vi "Generate PDF.vi"(8 "error in":errorcluster, 10 "Dynamic report parameters":T2, 11 "ZenReport private":T1) -> (0 "error out":errorcluster, 2 "Detailed error out":string, 3 "ZenReport private data":T1)   [LabVIEW 2015]
uses:
  Typedefs/Dynamic report parameters.ctl
  Typedefs/ZenReport private.ctl
  Typedefs/Report generation data cluster (internal use).ctl
  <vilib>/vision/Image Controls.llb/IMAQ Image.ctl
  <userlib>/_OpenG.lib/file/file.llb/Valid Path - Traditional__ogtk.vi
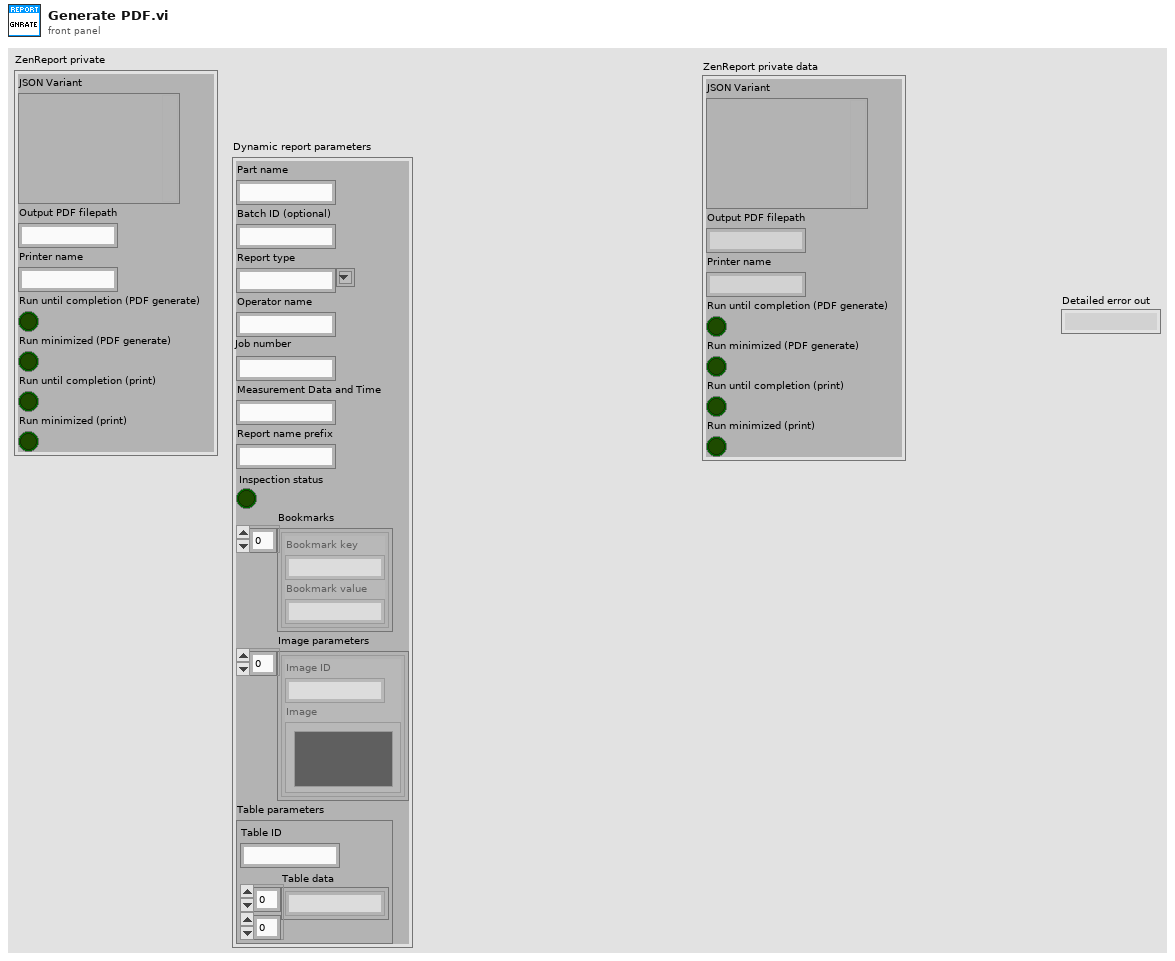
[diagram p1: front panel]
types:
  T1 = typedef "ZenReport private.ctl" = cluster{"JSON Variant":variant, "Output PDF filepath":string, "Printer name":string, "Run until completion (PDF generate)":bool, "Run minimized (PDF generate)":bool, "Run until completion (print)":bool, "Run minimized (print)":bool}
  T2 = typedef "Dynamic report parameters.ctl" = cluster{"Part name":string, "Batch ID (optional)":string, "Report type":string, "Operator name":string, "Job number":string, "Measurement Data and Time":string, "Report name prefix":string, "Inspection status":bool, "Bookmarks":cluster{"Bookmark key":string, "Bookmark value":string}[], "Image parameters":cluster{"Image ID":string, "Image":T3}[], "Table parameters":cluster{"Table ID":string, "Table data":string[][]}}
  T3 = typedef "IMAQ Image.ctl" = refnum<image>
  T4 = typedef "Report generation data cluster (internal use).ctl" = cluster{"Report data":cluster{"$part_name$":string, "$batch_id$":string, "$customer_name$":string, "$operator_name$":string, "$system_name$":string, "$measurement_date_and_time$":string, "$location$":string, "$job_number$":string, "$department$":string, "$status$":string, "Table details":string[][], "Output PDF filepath":string, "Output PDF folder filepath":path}, "Image details":cluster{"Image":T3, "Image filepath":path, "Use default scaling":bool, "Image scaling":cluster{"$image_width$":u32, "$image_height$":u32, "Unit":string}, "Resample factor":dbl}, "Report parameters":cluster{"Report auto name":bool, "Name prefix":string, "Printer name":string}}
  T5 = typedef "ZenReport internal data.ctl" = cluster{"ZenReport configuration":cluster{"System configuration":T6, "Part configuration":T7, "Batch parameters":T8}, "Report private parameters":T9}
  T6 = typedef "System configuration.ctl" = cluster{"System based configuration":cluster{"SystemName":string, "CompanyName":string, "Location":string, "Department":string, "LogoFilepath":string, "ImageTempFilePath":string, "PrinterParameters":cluster{"PrinterNamesList":string[], "DefaultPrinterName":string}}}
  T7 = typedef "Part configuration.ctl" = cluster{"Part configuration":cluster{"ReportType":string, "TableParameters":cluster{"TableID":dbl, "Column details":cluster{"ColumnName":string, "ColumnWidth":dbl, "ColumnTextAlignment":string}[]}[], "ImageParameters":cluster{"ImageID":string, "ImageBookmark":string, "ImageScalingParameters":cluster{"Width":u32, "Height":u32, "Unit":string}, "DefaultDisplayString":string, "ImageFilepath":string, "ResamplingFactor":dbl, "UseDefaultScaling":bool}[], "OutputReportNamePrefix":string, "OutputFilePath":string, "DefaultBookmarkValues":cluster{"BookmarkKey":string, "BookmarkValue":string}[]}}
  T8 = typedef "Batch configuration.ctl" = cluster{"Batch parameters":cluster{"ReportType":string, "TableParameters":cluster{"TableID":dbl, "Column details":cluster{"ColumnName":string, "ColumnWidth":dbl, "ColumnTextAlignment":string}[]}[], "OutputReportNamePrefix":string, "OutputFilePath":string, "ImageParameters":cluster{"ImageID":string, "ImageBookmark":string, "ImageScalingParameters":cluster{"Width":u32, "Height":u32, "Unit":string}, "DefaultDisplayString":string, "ImageFilepath":string, "ResamplingFactor":dbl, "UseDefaultScaling":bool}[]}}
  T9 = typedef "Internal data.ctl" = cluster{"Tex string":string}
  T10 = cluster{"ImageID":string, "ImageBookmark":string, "ImageScalingParameters":cluster{"Width":u32, "Height":u32, "Unit":string}, "DefaultDisplayString":string, "ImageFilepath":string, "ResamplingFactor":dbl, "UseDefaultScaling":bool}[]
  T11 = cluster{"ImageID":string, "ImageBookmark":string, "ImageScalingParameters":cluster{"Width":u32, "Height":u32, "Unit":string}, "DefaultDisplayString":string, "ImageFilepath":string, "ResamplingFactor":dbl, "UseDefaultScaling":bool}
  T12 = cluster{"Image":T3, "Image filepath":path, "Use default scaling":bool, "Image scaling":cluster{"$image_width$":u32, "$image_height$":u32, "Unit":string}, "Resample factor":dbl}
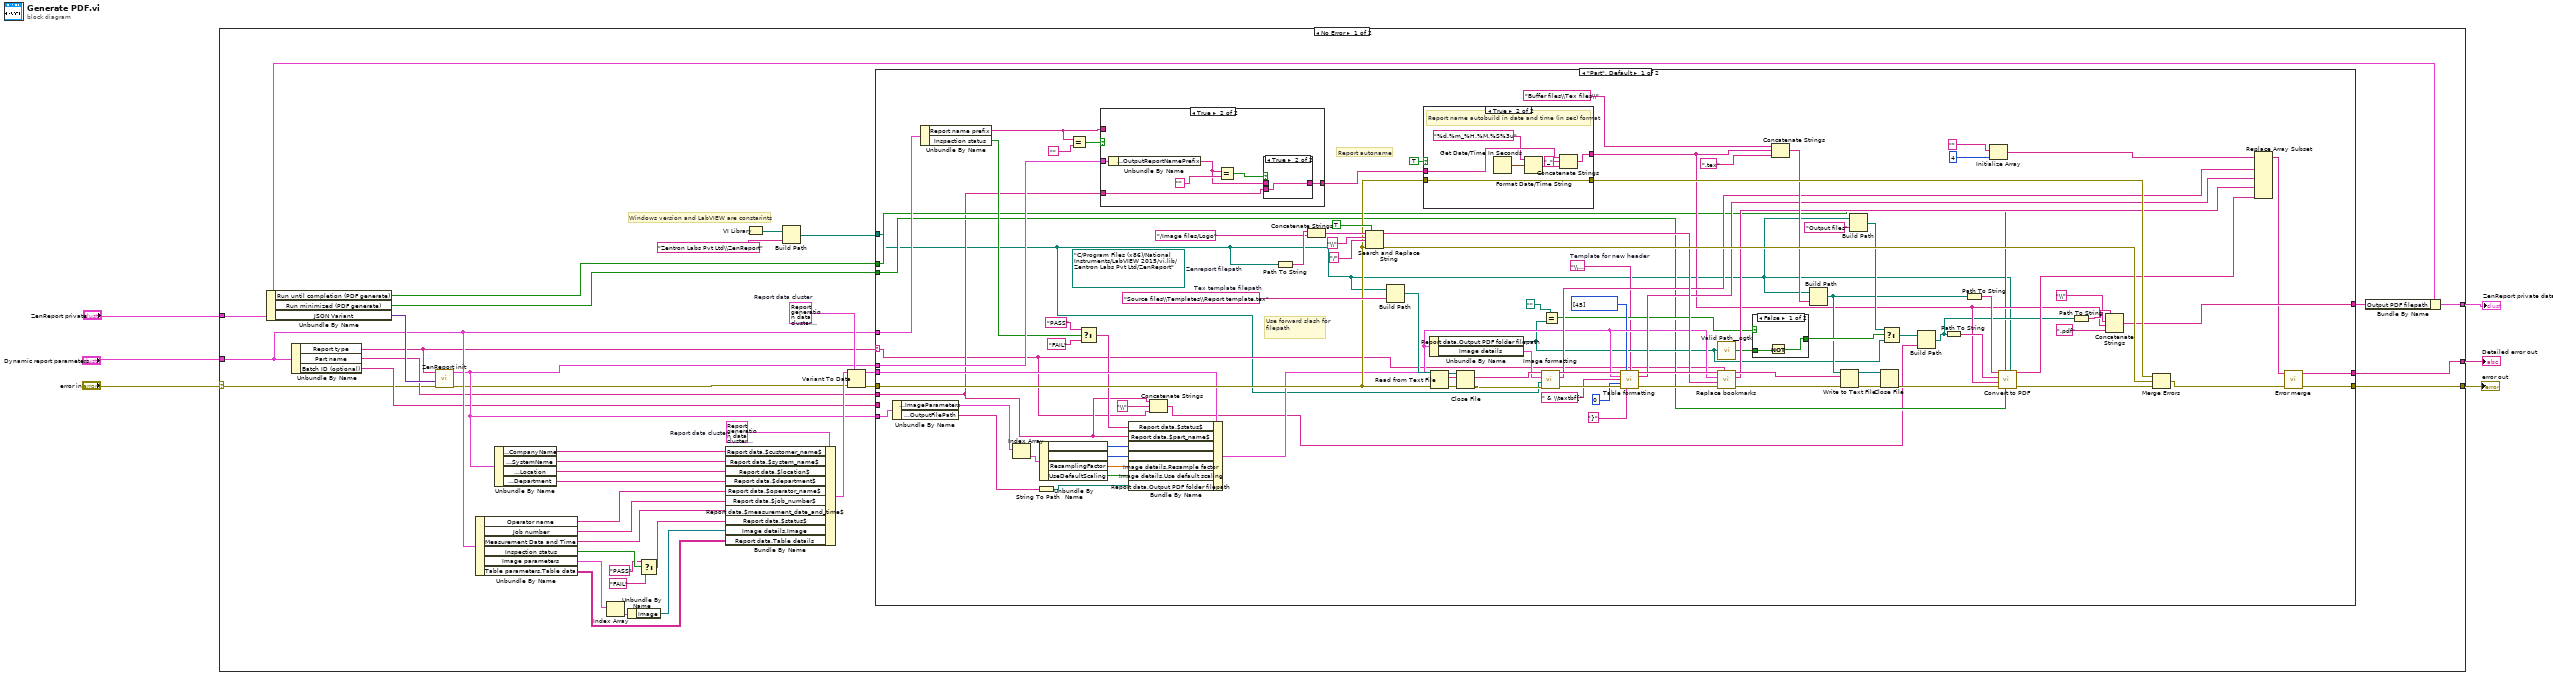
[diagram p0: block diagram]
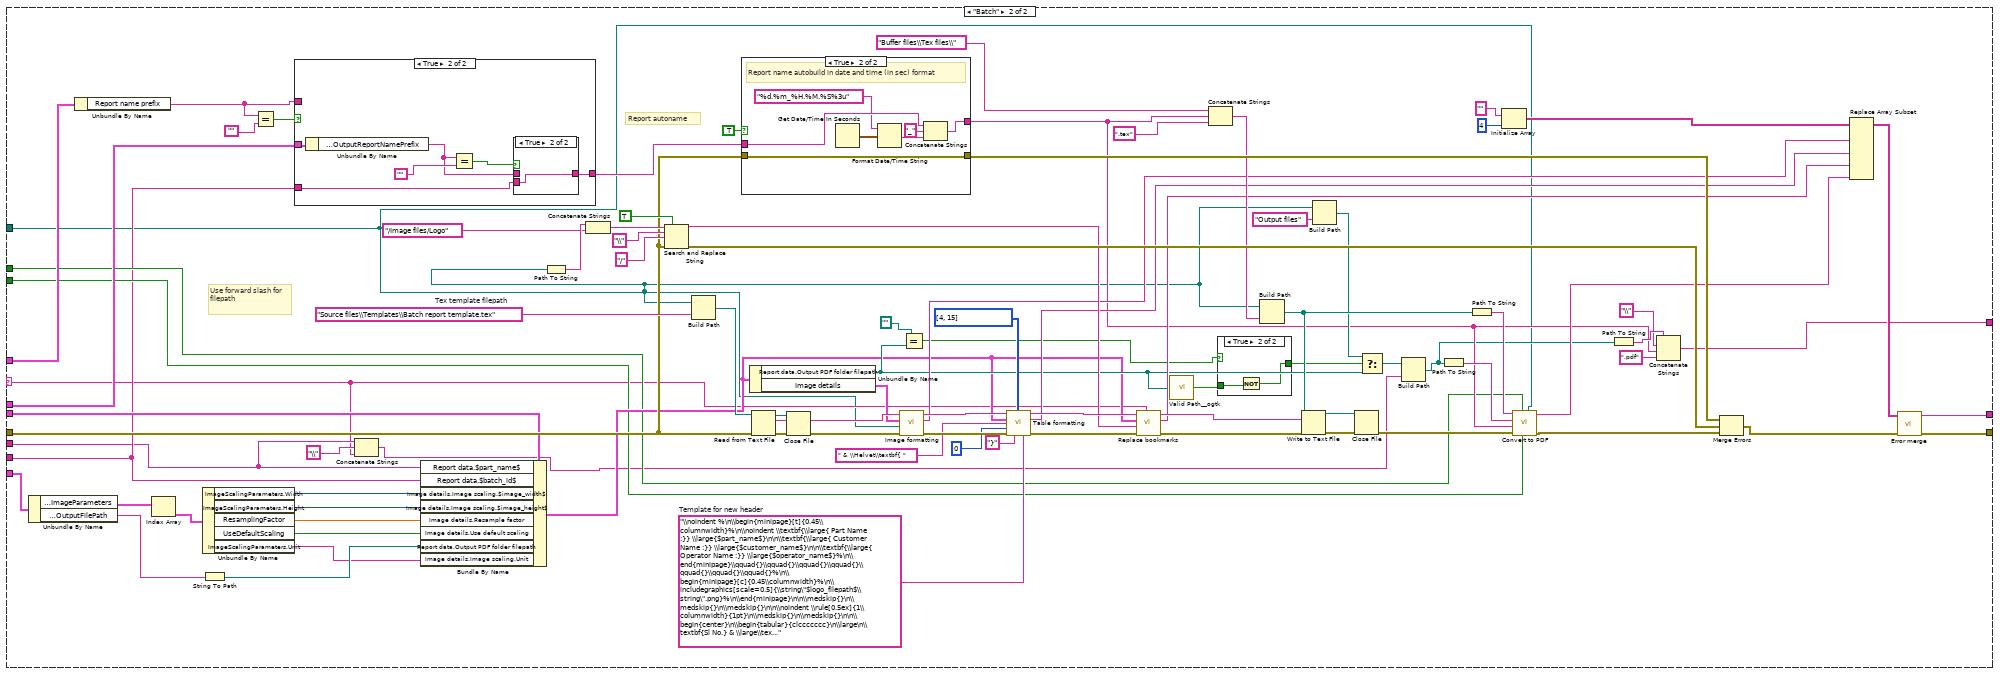
[diagram p6: hidden frame]
diagram:
  n1 = case shown="No Error" "error in" {
    selector: "error in" -> [w9 w267]
    tunnel: [w44 w267] -> w6
    tunnel: "Dynamic report parameters" -> [w25 _]
    tunnel: "ZenReport private" -> [w22 _]
    tunnel: [w11 _] -> w3
    tunnel: [w10 _] -> w2
    frame No Error {
      w27 = T4 {"Report data"={"$part_name$"="", "$batch_id$"="", "$customer_name$"="", "$operator_name$"="", "$system_name$"="", "$measurement_date_and_time$"="", "$location$"="", "$job_number$"="", "$department$"="", "$status$"="", "Table details"=[], "Output PDF filepath"="", "Output PDF folder filepath"=path ""}, "Image details"={"Image"=refnum, "Image filepath"=path "", "Use default scaling"=TRUE, "Image scaling"={"$image_width$"=0, "$image_height$"=0, "Unit"="mm"}, "Resample factor"=0.0}, "Report parameters"={"Report auto name"=FALSE, "Name prefix"="", "Printer name"=""}}  # Report data cluster
      w28 = T4 {"Report data"={"$part_name$"="", "$batch_id$"="", "$customer_name$"="", "$operator_name$"="", "$system_name$"="", "$measurement_date_and_time$"="", "$location$"="", "$job_number$"="", "$department$"="", "$status$"="", "Table details"=[], "Output PDF filepath"="", "Output PDF folder filepath"=path ""}, "Image details"={"Image"=refnum, "Image filepath"=path "", "Use default scaling"=TRUE, "Image scaling"={"$image_width$"=0, "$image_height$"=0, "Unit"="mm"}, "Resample factor"=0.0}, "Report parameters"={"Report auto name"=FALSE, "Name prefix"="", "Printer name"=""}}  # Report data cluster
      # "Windows version and LabVIEW are constarints"
      n2 = Unbundle By Name(w22) -> ("Run until completion (PDF generate)"=w15:bool, "Run minimized (PDF generate)"=w14:bool, "JSON Variant"=w43:variant)
      n3 = Unbundle By Name(w25) -> ("Report type"=w12:string, "Part name"=w13:string, "Batch ID (optional)"=w19:string)
      n4 = call "ZenReport init.vi"("error IO"=w9, "Get part / batch data"=w43, "Report type"=w12) -> ("Error out"=w8:errorcluster, "output cluster"=w20:T5)  [unwired: 7 in]
      n5 = Unbundle By Name(w25) -> ("Operator name"=w33:string, "Job number"=w34:string, "Measurement Data and Time"=w38:string, "Inspection status"=w37:bool, "Image parameters"=w40:cluster{"Image ID":string, "Image":T3}[], "Table parameters.Table data"=w7:string[][])
      n6 = Unbundle By Name(w20) -> ("ZenReport configuration.System configuration.System based configuration.CompanyName"=w29:string, "ZenReport configuration.System configuration.System based configuration.SystemName"=w30:string, "ZenReport configuration.System configuration.System based configuration.Location"=w31:string, "ZenReport configuration.System configuration.System based configuration.Department"=w32:string)
      n7 = Index Array(array=w40) -> (element=w41:cluster{"Image ID":string, "Image":T3})  [unwired: 1 in]
      n8 = Unbundle By Name(w41) -> ("Image"=w42:T3)
      n9 = Select(t="PASS", s=w37, f="FAIL") -> (s? t:f=w39:string)
      n10 = Bundle By Name(cluster=w28, "Report data.$customer_name$"=w29, "Report data.$system_name$"=w30, "Report data.$location$"=w31, "Report data.$department$"=w32, "Report data.$operator_name$"=w33, "Report data.$job_number$"=w34, "Report data.$measurement_date_and_time$"=w38, "Report data.$status$"=w39, "Image details.Image"=w42, "Report data.Table details"=w7) -> (w26:T4)
      n11 = VI Library() -> (path=w18:path)
      n12 = Build Path(base path=w18, name or relative path="Zentron Labs Pvt Ltd\\ZenReport") -> (appended path=w16:path)
      n13 = Variant To Data(error in=w8, type=w27, Variant=w26) -> (data=w23:T4, error out=w24:errorcluster)
      n14 = case shown="\"Part\", Default" w12 {
        selector: w12 -> [w47 w159]
        tunnel: [w51 w163] -> w44
        tunnel: [w91 w199] -> w10
        tunnel: w24 -> [w89 w196]
        tunnel: w20 -> [w64 w193]
        tunnel: w25 -> [w63 w173]
        tunnel: w16 -> [w45 w157]
        tunnel: w23 -> [w80 w175]
        tunnel: [w88 w192] -> w21
        tunnel: w20 -> [w76 w189]
        tunnel: w13 -> [w48 w161]
        tunnel: w19 -> [_ w162]
        tunnel: w15 -> [w53 w165]
        tunnel: w14 -> [w52 w164]
        frame "Part", Default {
          w61 = "\\noindent %\n\\begin{minipage}[t]{0.45\\columnwidth}%\n\\noindent \\textbf{Part Name : $part_name$}\n\n\\textbf{Customer Name : $customer_name$}\n\n\\textbf{Operator Name : $operator_name$}%\n\\end{minipage}\\qquad{}\\qquad{}\\qquad{}\\qquad{}\\qquad{}\\qquad{}\\qquad{}%\n\\begin{minipage}[c]{0.45\\columnwidth}%\n\\includegraphics[scale=0.5]{\\string\"$logo_filepath$\\string\".png}%\n\\end{minipage}\n\n\\medskip{}\n\\medskip{}\n\\medskip{}\n\n\\noindent \\rule[0.5ex]{1\\columnwidth}{1pt}\n\n\\begin{center}\n\\begin{tabular}{clccccccc}\n\\textbf{SL.NO} & \\textbf{DESCRIPTION} & \\textbf{LSL} & \\textbf{NOMINAL} & \\textbf{USL} & \\textbf{MEASURED} & \\textbf{DEVIATION} & \\textbf{UNITS} & \\textbf{STATUS}\\tabularnewline\n &  &  &  &  &  &  &  & \\tabularnewline\n$table2$\n\\end{tabular}\n\\end{center}\n\n\\end{document}\n"  # Template for new header
          (unwired) path "C:/Program Files (x86)/National Instruments/LabVIEW 2015/vi.lib/Zentron Labs Pvt Ltd/ZenReport"  # Zenreport filepath
          w135 = "Source files\\Templates\\Report template.tex"  # Tex template filepath
          # "Report autoname"
          # "Use forward slash for filepath"
          n15 = Unbundle By Name(w76) -> ("ZenReport configuration.Part configuration.Part configuration.ImageParameters"=w75:T10, "ZenReport configuration.Part configuration.Part configuration.OutputFilePath"=w73:string)
          n16 = Unbundle By Name(w63) -> ("Report name prefix"=w65:string, "Inspection status"=w58:bool)
          n17 = Index Array(array=w75) -> (element=w84:T11)  [unwired: 1 in]
          n18 = String To Path(string=w73) -> (path=w74:path)
          n19 = Unbundle By Name(w84) -> ("ImageScalingParameters.Width"=w83:u32, "ImageScalingParameters.Height"=w82:u32, "ResamplingFactor"=w81:dbl, "UseDefaultScaling"=w78:bool)
          n20 = Equal?(x=w65, y="") -> (x = y?=w66:bool)
          n21 = Select(t="PASS", s=w58, f="FAIL") -> (s? t:f=w57:string)
          n22 = case shown="True" w66 {
            tunnel: [w136 w140] -> w62
            tunnel: w64 -> [_ w138]
            tunnel: w48 -> [_ w137]
            tunnel: w65 -> [w136 _]
            frame False {
            }
            frame True {
              n23 = Unbundle By Name(w138) -> ("ZenReport configuration.Part configuration.Part configuration.OutputReportNamePrefix"=w139:string)
              n24 = Equal?(x=w139, y="") -> (x = y?=w141:bool)
              n25 = case shown="True" w141 {
                tunnel: [w143 w144] -> w140
                tunnel: w139 -> [w143 _]
                tunnel: w137 -> [_ w144]
                frame False {
                }
                frame True {
                }
              }
            }
          }
          n26 = Bundle By Name(cluster=w80, "Report data.$status$"=w57, "Report data.$part_name$"=w48, "Image details.Image scaling.$image_width$"=w83, "Image details.Image scaling.$image_height$"=w82, "Image details.Resample factor"=w81, "Image details.Use default scaling"=w78, "Report data.Output PDF folder filepath"=w74) -> (w79:T4)
          n27 = Concatenate Strings(w48, "\\" ("string"), w47) -> (w46:string)
          n28 = Path To String(path=w45) -> (string=w129:string)
          n29 = Concatenate Strings(w129, "/Image files/Logo") -> (w127:string)
          n30 = Search and Replace String(replace all?=TRUE ("replace all? (F)"), input string=w127, search string="\\", replace string="/" ("replace string (\"\")"), error in=w89) -> (result string=w106:string, error out=w123:errorcluster)  [unwired: 3 in, 2 out]
          n31 = Build Path(base path=w45, name or relative path=w135) -> (appended path=w134:path)
          n32 = case shown="True" TRUE {
            tunnel: w62 -> [w149 w154]
            tunnel: [w149 w155] -> w56
            tunnel: w89 -> [w148 w152]
            tunnel: [w148 w152] -> w119
            frame False {
              # "Write in given name"
            }
            frame True {
              # "Report name autobuild in date and time (in sec) format"
              n33 = Get Date/Time In Seconds() -> (seconds since 1Jan1904=w156:timestamp)
              n34 = Format Date/Time String(time format string (%c)="%d.%m_%H.%M.%S%3u", seconds (now)=w156) -> (date/time string=w150:string)  [unwired: 1 in]
              n35 = Concatenate Strings(w154, "_" ("string"), w150) -> (w155:string)
            }
          }
          n36 = Unbundle By Name(w79) -> ("Report data.Output PDF folder filepath"=w68:path, "Image details"=w112:T12)
          n37 = Read from Text File(file (use dialog)=w134, error in=w89) -> (refnum out=w131:refnum<file>, text=w113:string, error out=w132:errorcluster)  [unwired: 2 in, 1 out]
          n38 = Close File(refnum=w131, error in=w132) -> (error out=w114:errorcluster)  [unwired: 1 out]
          n39 = call "Image formatting.vi"("error in (no error)"=w114, "Zenreport filepath"=w45, "Image details"=w112, "Tex string in"=w113) -> ("error out"=w122:errorcluster, "Error details out"=w94:string, "Tex string out"=w111:string)  [unwired: 5 in]
          n40 = Equal?(x=path "", y=w68) -> (x = y?=w72:bool)
          n41 = call "Table formatting.vi"("Input tex string"=w111, "Table row count array"=i32[] [45], "Template for new header"=w61, "Report data cluster"=w79, "Separator"=" & \\textbf{", "Iteration count"=u8 0, "error in (no error)"=w122, "End tag"="}") -> ("Tex string out"=w108:string, "Error details out"=w93:string, "error out"=w110:errorcluster)  [unwired: 5 in]
          n42 = call "Replace bookmarks.vi"("Report type"=w47, "error in (no error)"=w110, "Logo filepath"=w106, "Report data cluster"=w79, "Tex file string"=w108) -> ("error out"=w109:errorcluster, "Error detail out"=w92:string, "Tex file string out"=w107:string)  [unwired: 4 in]
          n43 = call-poly <userlib>:"Valid Path__ogtk.vi"("path"=w68) -> ("valid"=w71:bool)
          n44 = case shown="False" w72 {
            selector: w72 -> [_ w147]
            tunnel: w71 -> [w146 _]
            tunnel: [w145 w147] -> w70
            frame False {
              n45 = Not(x=w146) -> (.not. x?=w145:bool)
            }
            frame True {
            }
          }
          n46 = Concatenate Strings("Buffer files\\Tex files\\" ("string"), w56, ".tex" ("string")) -> (w118:string)
          n47 = Build Path(base path=w45, name or relative path=w118) -> (appended path=w69:path)
          n48 = Write to Text File(file (use dialog)=w69, text=w107, error in=w109) -> (refnum out=w130:refnum<file>, error out=w133:errorcluster)  [unwired: 1 in, 1 out]
          n49 = Build Path(base path=w45, name or relative path="Output files") -> (appended path=w100:path)
          n50 = Close File(refnum=w130, error in=w133) -> (error out=w105:errorcluster)  [unwired: 1 out]
          n51 = Select(t=w100, s=w70, f=w68) -> (s? t:f=w55:path)
          n52 = Build Path(base path=w55, name or relative path=w46) -> (appended path=w54:path)
          n53 = Path To String(path=w54) -> (string=w99:string)
          n54 = Path To String(path=w69) -> (string=w103:string)
          n55 = Initialize Array("", 4 ("dimension size")) -> (w96:string[])
          n56 = call "Convert to PDF.vi"("Zenreport filepath"=w45, "run minimized? (F)"=w52, "wait until completion? (T)"=w53, "error in"=w105, "PDF name"=w56, "Destination filepath"=w99, "Source filepath"=w103) -> ("error out"=w104:errorcluster, "Error detail out"=w95:string)  [unwired: 3 in]
          n57 = Path To String(path=w54) -> (string=w116:string)
          n58 = Concatenate Strings(w116, "\\" ("string"), w56, ".pdf" ("string")) -> (w88:string)
          n59 = Merge Errors(w119, w123, w104) -> (w51:errorcluster)
          n60 = Replace Array Subset(array=w96, new element #1=w94, new element #2=w93, new element #3=w92, new element #4=w95) -> (w50:string[])  [unwired: 4 in]
          n61 = call "Error merge.vi"("Error details array"=w50) -> ("Detailed error out"=w91:string)  [unwired: 10 in]
        }
        frame "Batch" {
          w169 = "\\noindent %\n\\begin{minipage}[t]{0.45\\columnwidth}%\n\\noindent \\textbf{\\large{ Part Name :}} \\large{$part_name$}\n\n\\textbf{\\large{ Customer Name :}} \\large{$customer_name$}\n\n\\textbf{\\large{ Operator Name :}} \\large{$operator_name$}%\n\\end{minipage}\\qquad{}\\qquad{}\\qquad{}\\qquad{}\\qquad{}\\qquad{}\\qquad{}%\n\\begin{minipage}[c]{0.45\\columnwidth}%\n\\includegraphics[scale=0.5]{\\string\"$logo_filepath$\\string\".png}%\n\\end{minipage}\n\n\\medskip{}\n\\medskip{}\n\\medskip{}\n\n\\noindent \\rule[0.5ex]{1\\columnwidth}{1pt}\n\\medskip{}\n\\medskip{}\n\n\\begin{center}\n\\begin{tabular}{clccccccc}\n\\large\n\\textbf{Sl No.} & \\large\\textbf{Measurement Name} & \\large\\textbf{Mean} & \\large\\textbf{Variance} & \\large\\textbf{Standard deviation} & \\large\\textbf{Cp} & \\large\\textbf{Cpk}\\tabularnewline\n &  &  &  &  &  &  &  & \\tabularnewline\n$table2$\n\n\\end{tabular}\n\\end{center}\n\\end{document}\n"  # Template for new header
          w245 = "Source files\\Templates\\Batch report template.tex"  # Tex template filepath
          # "Report autoname"
          # "Use forward slash for filepath"
          n62 = Unbundle By Name(w189) -> ("ZenReport configuration.Batch parameters.Batch parameters.ImageParameters"=w187:T10, "ZenReport configuration.Batch parameters.Batch parameters.OutputFilePath"=w182:string)
          n63 = Unbundle By Name(w173) -> ("Report name prefix"=w170:string)
          n64 = Index Array(array=w187) -> (element=w188:T11)  [unwired: 1 in]
          n65 = Unbundle By Name(w188) -> ("ImageScalingParameters.Width"=w186:u32, "ImageScalingParameters.Height"=w185:u32, "ResamplingFactor"=w184:dbl, "UseDefaultScaling"=w183:bool, "ImageScalingParameters.Unit"=w176:string)
          n66 = String To Path(string=w182) -> (path=w177:path)
          n67 = Equal?(x=w170, y="") -> (x = y?=w171:bool)
          n68 = case shown="True" w171 {
            tunnel: [w246 w250] -> w198
            tunnel: w193 -> [_ w248]
            tunnel: w162 -> [_ w247]
            tunnel: w170 -> [w246 _]
            frame False {
            }
            frame True {
              n69 = Unbundle By Name(w248) -> ("ZenReport configuration.Part configuration.Part configuration.OutputReportNamePrefix"=w249:string)
              n70 = Equal?(x=w249, y="") -> (x = y?=w251:bool)
              n71 = case shown="True" w251 {
                tunnel: [w253 w254] -> w250
                tunnel: w249 -> [w253 _]
                tunnel: w247 -> [_ w254]
                frame False {
                }
                frame True {
                }
              }
            }
          }
          n72 = Concatenate Strings(w161, "\\" ("string"), w159) -> (w158:string)
          n73 = Bundle By Name(cluster=w175, "Report data.$part_name$"=w161, "Report data.$batch_id$"=w162, "Image details.Image scaling.$image_width$"=w186, "Image details.Image scaling.$image_height$"=w185, "Image details.Resample factor"=w184, "Image details.Use default scaling"=w183, "Report data.Output PDF folder filepath"=w177, "Image details.Image scaling.Unit"=w176) -> (w174:T4)
          n74 = Path To String(path=w157) -> (string=w238:string)
          n75 = Concatenate Strings(w238, "/Image files/Logo") -> (w236:string)
          n76 = Search and Replace String(replace all?=TRUE ("replace all? (F)"), input string=w236, search string="\\", replace string="/" ("replace string (\"\")"), error in=w196) -> (result string=w215:string, error out=w232:errorcluster)  [unwired: 3 in, 2 out]
          n77 = Build Path(base path=w157, name or relative path=w245) -> (appended path=w244:path)
          n78 = case shown="True" TRUE {
            tunnel: w198 -> [w259 w264]
            tunnel: [w259 w265] -> w168
            tunnel: w196 -> [w258 w262]
            tunnel: [w258 w262] -> w228
            frame False {
              # "Write in given name"
            }
            frame True {
              # "Report name autobuild in date and time (in sec) format"
              n79 = Get Date/Time In Seconds() -> (seconds since 1Jan1904=w266:timestamp)
              n80 = Format Date/Time String(time format string (%c)="%d.%m_%H.%M.%S%3u", seconds (now)=w266) -> (date/time string=w260:string)  [unwired: 1 in]
              n81 = Concatenate Strings(w264, "_" ("string"), w260) -> (w265:string)
            }
          }
          n82 = Unbundle By Name(w174) -> ("Report data.Output PDF folder filepath"=w181:path, "Image details"=w221:T12)
          n83 = Read from Text File(file (use dialog)=w244, error in=w196) -> (refnum out=w241:refnum<file>, text=w222:string, error out=w242:errorcluster)  [unwired: 2 in, 1 out]
          n84 = Close File(refnum=w241, error in=w242) -> (error out=w223:errorcluster)  [unwired: 1 out]
          n85 = call "Image formatting.vi"("error in (no error)"=w223, "Zenreport filepath"=w157, "Image details"=w221, "Tex string in"=w222) -> ("error out"=w231:errorcluster, "Error details out"=w203:string, "Tex string out"=w220:string)  [unwired: 5 in]
          n86 = Equal?(x=path "", y=w181) -> (x = y?=w179:bool)
          n87 = call "Table formatting.vi"("Input tex string"=w220, "Table row count array"=i32[] [4, 15], "Template for new header"=w169, "Report data cluster"=w174, "Separator"=" & \\Helvet\\textbf{ ", "Iteration count"=u8 0, "error in (no error)"=w231, "End tag"="}") -> ("Tex string out"=w217:string, "Error details out"=w202:string, "error out"=w219:errorcluster)  [unwired: 5 in]
          n88 = call "Replace bookmarks.vi"("Report type"=w159, "error in (no error)"=w219, "Logo filepath"=w215, "Report data cluster"=w174, "Tex file string"=w217) -> ("error out"=w218:errorcluster, "Error detail out"=w201:string, "Tex file string out"=w216:string)  [unwired: 4 in]
          n89 = call-poly <userlib>:"Valid Path__ogtk.vi"("path"=w181) -> ("valid"=w180:bool)
          n90 = Concatenate Strings("Buffer files\\Tex files\\" ("string"), w168, ".tex" ("string")) -> (w227:string)
          n91 = case shown="True" w179 {
            selector: w179 -> [w255 _]
            tunnel: w180 -> [_ w257]
            tunnel: [w255 w256] -> w178
            frame False {
            }
            frame True {
              n92 = Not(x=w257) -> (.not. x?=w256:bool)
            }
          }
          n93 = Build Path(base path=w157, name or relative path=w227) -> (appended path=w239:path)
          n94 = Write to Text File(file (use dialog)=w239, text=w216, error in=w218) -> (refnum out=w240:refnum<file>, error out=w243:errorcluster)  [unwired: 1 in, 1 out]
          n95 = Build Path(base path=w157, name or relative path="Output files") -> (appended path=w209:path)
          n96 = Close File(refnum=w240, error in=w243) -> (error out=w214:errorcluster)  [unwired: 1 out]
          n97 = Select(t=w209, s=w178, f=w181) -> (s? t:f=w167:path)
          n98 = Build Path(base path=w167, name or relative path=w158) -> (appended path=w166:path)
          n99 = Path To String(path=w166) -> (string=w208:string)
          n100 = Path To String(path=w239) -> (string=w212:string)
          n101 = Initialize Array("", 4 ("dimension size")) -> (w205:string[])
          n102 = call "Convert to PDF.vi"("Zenreport filepath"=w157, "run minimized? (F)"=w164, "wait until completion? (T)"=w165, "error in"=w214, "PDF name"=w168, "Destination filepath"=w208, "Source filepath"=w212) -> ("error out"=w213:errorcluster, "Error detail out"=w204:string)  [unwired: 3 in]
          n103 = Path To String(path=w166) -> (string=w225:string)
          n104 = Concatenate Strings(w225, "\\" ("string"), w168, ".pdf" ("string")) -> (w192:string)
          n105 = Merge Errors(w228, w232, w213) -> (w163:errorcluster)
          n106 = Replace Array Subset(array=w205, new element #1=w203, new element #2=w202, new element #3=w201, new element #4=w204) -> (w200:string[])  [unwired: 4 in]
          n107 = call "Error merge.vi"("Error details array"=w200) -> ("Detailed error out"=w199:string)  [unwired: 10 in]
        }
      }
      n108 = Bundle By Name(cluster=w22, "Output PDF filepath"=w21) -> (w11:T1)
    }
    frame Error {
    }
  }
  "error out" <- w6
  "Detailed error out" <- w2
  "ZenReport private data" <- w3
